vi "voltage.vi"() -> ()   [LabVIEW 2015]
panel:
  in  "stop":bool
  out "Numeric 3":dbl format="%#.4g"
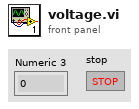
[diagram p1: front panel]
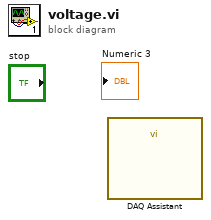
[diagram p0: block diagram]
diagram:
  n1 = call "DAQ Assistant"() -> ()  [unwired: 17 in, 3 out]
